vi "SR430.set records per scan.vi"(0 "i ref in":refnum<vi>, 2 "records per scan":i32, 5 "error in (no error)":errorcluster) -> (14 "i ref out":refnum<vi>, 19 "error out":errorcluster)   [LabVIEW 2014, in "SR430.lvlib"]
doc: "Sets the record per scan at the SR430. This is the number of records that will be accumulated. The number of records ranges from 0 to 65535. When set to 0, accumulation will continue indefinitely."
uses:
  SR430.lvlib
  CS_Core/CSApplicationBaseClasses/MCSBase/MCSBase.directionType.ctl
  CS_Core/CSApplicationBaseClasses/MCSBase/MCSBase.serviceType.ctl
  CSlibraries/UtilityLib/UtilityLib.valueStatus.ctl
  CS_Core/CSSystem/CoreDefs/CoreDefs.error_type.ctl
  instr.lib/SR430/SR430Driver.lvlib
  CS_Core/CSSystem/CoreLib/CoreLib.lvlib
  CS_Core/CSApplicationBaseClasses/MCSBase/MCSBase.lvlib
  CSlibraries/UtilityLib/UtilityLib.lvlib
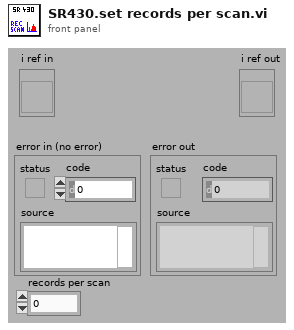
[diagram p1: front panel]
types:
  T1 = typedef "UtilityLib.lvlib/UtilityLib.valueStatus.ctl" = enum16{"no info available", "stand by/off", "on", "warning", "alarm/malfunction", "not implemented", "user action required", "important information", "system default", "control default", "indicator default", "button default"}
  T2 = typedef "MCSBase.lvlib/MCSBase.serviceType.ctl" = enum16{"counts", "totalCounts", "binWidth", "nOfBins", "nOfRecords", "status", "discrLevel", "discrSlope", "triggerLevel", "triggerSlope"}
  T3 = typedef "MCSBase.lvlib/MCSBase.directionType.ctl" = enum16{"unknown", "update actual value", "update nominal value", "update both"}
  T4 = typedef "CoreDefs.error_type.ctl" = enum16{"no error", "can't load process", "can't unload process", "process does not exist", "can't install process", "can't remove process", "unknown function", "time out", "can't execute function", "duplicate queue name", "super not found", "caller queue invalid", "can't ping process", "unknown error", "VISA Error", "VISA timeout", "GPIB timeout", "GPIB error", "communication error", "data type mismatch", "can't read data from OPC server", "can't write data to OPC server", "OET error", "function not implemented", "process already exists", "invalid Shared Variable name", "error writing Shared Variable", "error reading Shared Variable", "invalid client name", "corrupt database", "unknown class", "call not authorized", "parameter out of range", "OET timeout: can't get data to modify", "invalid queue name", "requested operation incompatible with current state", "event undefined", "event disabled", "state undefined", "caller is not a friend", "EventBuilder: bad eventID", "EventBuilder: no DAQ devices", "a thread must not stop itself", "UNUSED ELEMENT4", "DiscArchiver: eventData incomplete", "DiscArchiver: eventData does not belong to run", "DiscArchiver: can't open file", "DiscArchiver: can't write to file", "DiscArchiver: available disc space low", "can't acquire semaphore", "error reading data from database", "notifier object is not existing", "can't register process", "can't unregister process", "illegal event type", "object disabled", "object already exists", "can't change state", "Instrument not found", "no connection to remote node", "invalid reference", "N/A", "UNUSED ELEMENT 1", "element not found", "illegal TCP/IP connection detected", "object does not exist", "invalid access ID", "unknown CS system", "invalid privilige", "unsupported data type", "unsupported server type", "IO server already exists", "Shared Variable already exists"}
  T5 = typedef "SR430Driver.lvlib/SR430_VISA Control.ctl" = cluster{"VISA resource name":refnum<visa-resource-name>}
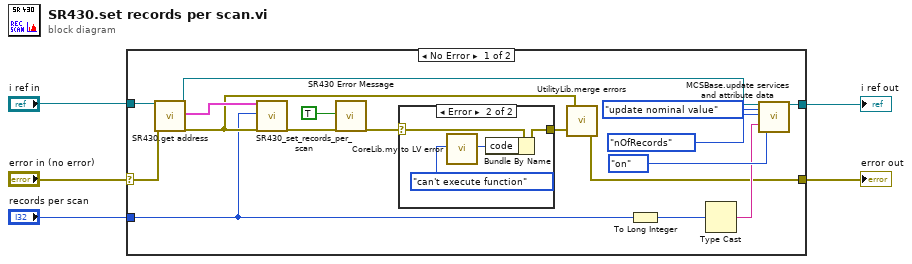
[diagram p0: block diagram]
diagram:
  n1 = case shown="No Error" "error in (no error)" {
    selector: "error in (no error)" -> [w15 w28]
    tunnel: "i ref in" -> [w22 w29]
    tunnel: "records per scan" -> [w7 _]
    tunnel: [w10 w28] -> w3
    tunnel: [w9 w29] -> w2
    frame No Error {
      n2 = call "SR430.get address.vi"("i ref in"=w22, "error in (no error)"=w15) -> ("i ref out"=w8:refnum<vi>, "address"=w21:T5, "error out"=w20:errorcluster)  [unwired: 15 in]
      n3 = call "SR430_set_records_per_scan.vi"("address string"=w21, "recordsPerScan"=w7, "error in (no error)"=w20) -> ("error out"=w19:errorcluster)  [unwired: 15 in, 1 out]
      n4 = call "SR430 Error Message.vi"("addMessageToSource"=TRUE ("add message to source"), "error in (no error)"=w19) -> ("error out"=w18:errorcluster)  [unwired: 14 in, 3 out]
      n5 = case shown="Error" w18 {
        selector: w18 -> [w23 w27]
        tunnel: [w23 w24] -> w16
        frame No Error {
        }
        frame Error {
          n6 = call "CoreLib.my to LV error.vi"("ErrorTypes"=CoreDefs.error_type."can't execute function") -> ("LV error code"=w26:i32)  [unwired: 17 in, 1 out]
          n7 = Bundle By Name(cluster=w27, "code"=w26) -> (w24:errorcluster)
        }
      }
      n8 = call "UtilityLib.merge errors.vi"("error2 (no error)"=w16, "error1 (no error)"=w20) -> ("error out"=w10:errorcluster)
      n9 = To Long Integer(number=w7) -> (32bit integer=w6:i32)
      n10 = Type Cast(x=w6) -> (*(type *) &x=w11:string)  [unwired: 1 in]
      n11 = call "MCSBase.update services and attribute data.vi"("i ref in"=w8, "direction"=MCSBase.directionType."update nominal value", "service"=MCSBase.serviceType."nOfRecords", "value"=w11, "quality"=UtilityLib.valueStatus."on") -> ("i ref out"=w9:refnum<vi>)  [unwired: 12 in, 2 out]
    }
    frame Error {
    }
  }
  "error out" <- w3
  "i ref out" <- w2
